vi "DetectOddEvenNum.vi"() -> ()   [LabVIEW 2024]
uses:
  <vilib>/numeric/Random Number (Range) U64.vi
  <vilib>/numeric/sub_Random U32.vi
panel:
  out "Even":bool
  out "Waveform Graph":u64[](graph)
  out "Array":dbl[](array[numeric])
  out "Waveform Chart":u64(graph)
  out "Odd":bool
  out "No of iteration":i32
  in  "milliseconds to wait":u32
  in  "No of loop":i32
  out "number":u64
  in  "lower bound (0)":u64
  in  "upper bound (100)":u64=100
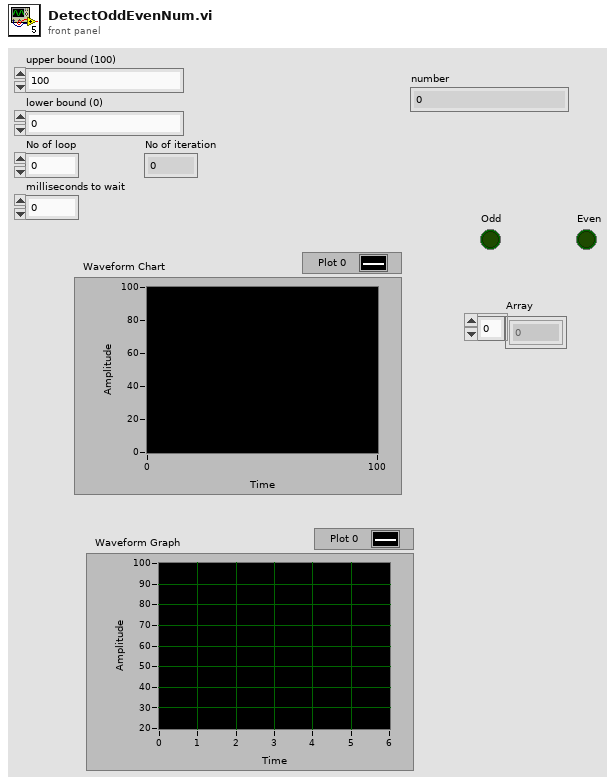
[diagram p1: front panel]
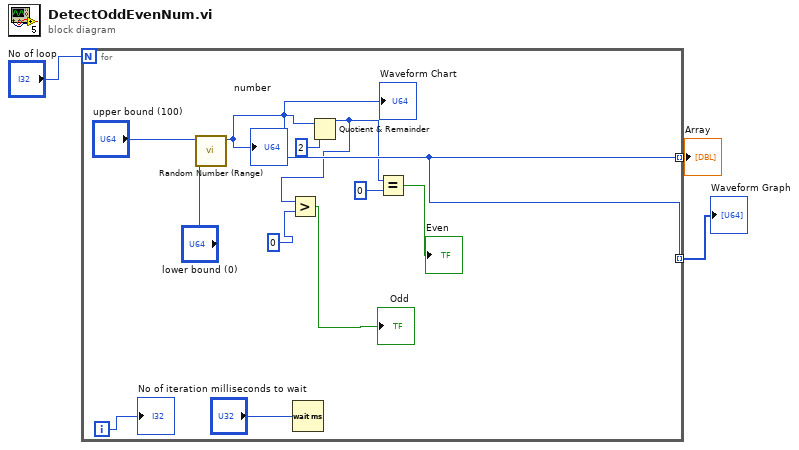
[diagram p0: block diagram]
diagram:
  n1 = for {
    N: "No of loop" -> [_]
    tunnel: [w9] -> w2 mode=indexing
    tunnel: [w9] -> w1 mode=indexing
    i -> [w11]
    n2 = call-poly <vilib>:"Random Number (Range).vi"("lower bound (0)"="lower bound (0)", "upper bound (100)"="upper bound (100)") -> ("number"=w9:u64)  [unwired: 9 in]
    "number" <- w9
    "Waveform Chart" <- w9
    n3 = Wait (ms)(milliseconds to wait="milliseconds to wait") -> ()  [unwired: 1 out]
    n4 = Quotient & Remainder(x=w9, y=2) -> (x-y*floor(x/y)=w4:u64)  [unwired: 1 out]
    n5 = Greater?(x=w4, y=0) -> (0:→"Odd":bool)
    n6 = Equal?(x=w4, y=u64 0) -> (x = y?=→"Even":bool)
    "No of iteration" <- w11
  }
  "Array" <- w2
  "Waveform Graph" <- w1
